vi "RT Loop - RSI Low Speed.vi"(11 "Message Queue":refnum<queue>) -> ()   [LabVIEW 2017]
doc: "This RSI Low Speed Loop VI acquires temperature data and digital inputs, and updates digital outputs."
uses:
  support/Message Queue/Message Cluster.ctl
  <vilib>/Platform/TimedLoop/XDataNode/timing_clust.ctl
  <vilib>/Platform/TimedLoop/XDataNode/nitl_modes.ctl
  <vilib>/Platform/TimedLoop/XDataNode/wakeup.ctl
  controls/Control State.ctl
  <vilib>/Platform/TimedLoop/XDataNode/loadnilvce.vi
  <vilib>/Platform/TimedLoop/XDataNode/XDataNode.xnode
  <vilib>/Platform/TimedLoop/XDataNode/XDNodeRunTimeDep.lvlib
  support/Message Queue/Message Queue.lvlib
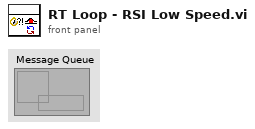
[diagram p1: front panel]
types:
  T1 = typedef "XDNodeRunTimeDep.lvlib/timing_clust.ctl" = cluster{"Expected End [f-1]":u64, "Actual End [f-1]":u64, "Finished Late? [f-1]":bool, "Expected End [i-1]":u64, "Actual End [i-1]":u64, "Finished Late? [i-1]":bool, "Expected Start [i]":u64, "Actual Start [i]":u64, "Expected Start [f]":u64, "Actual Start [f]":u64, "Source Name":string, "Structure Name":string, "Period":i64, "Deadline":i64, "Offset":i64, "Start":i64, "Priority":i32, "Timeout":i32, "Mode":T2, "Wakeup Reason":T3, "Error":errorcluster, "Source Type":string, "Secondary Source Type":string, "Global End Time":u64, "Global Start Time":u64, "Frame Duration":u64, "Iteration Duration":u64, "Assigned CPU":i32, "I/O Scan Engine Mode":u32}
  T2 = typedef "XDNodeRunTimeDep.lvlib/nitl_modes.ctl" = enum32{"No Change", "Process missed periods, maintain original phase", "Discard missed periods, maintain original phase", "Process missed periods, ignore original phase", "Discard missed periods, ignore original phase"}
  T3 = typedef "XDNodeRunTimeDep.lvlib/wakeup.ctl" = enum32{"Normal", "Aborted", "Asynchronous wakeup", "Timing source error", "Timed loop error", "Timeout"}
  T4 = typedef "Control State.ctl" = enum16{"Safe State", "Control (PID)"}
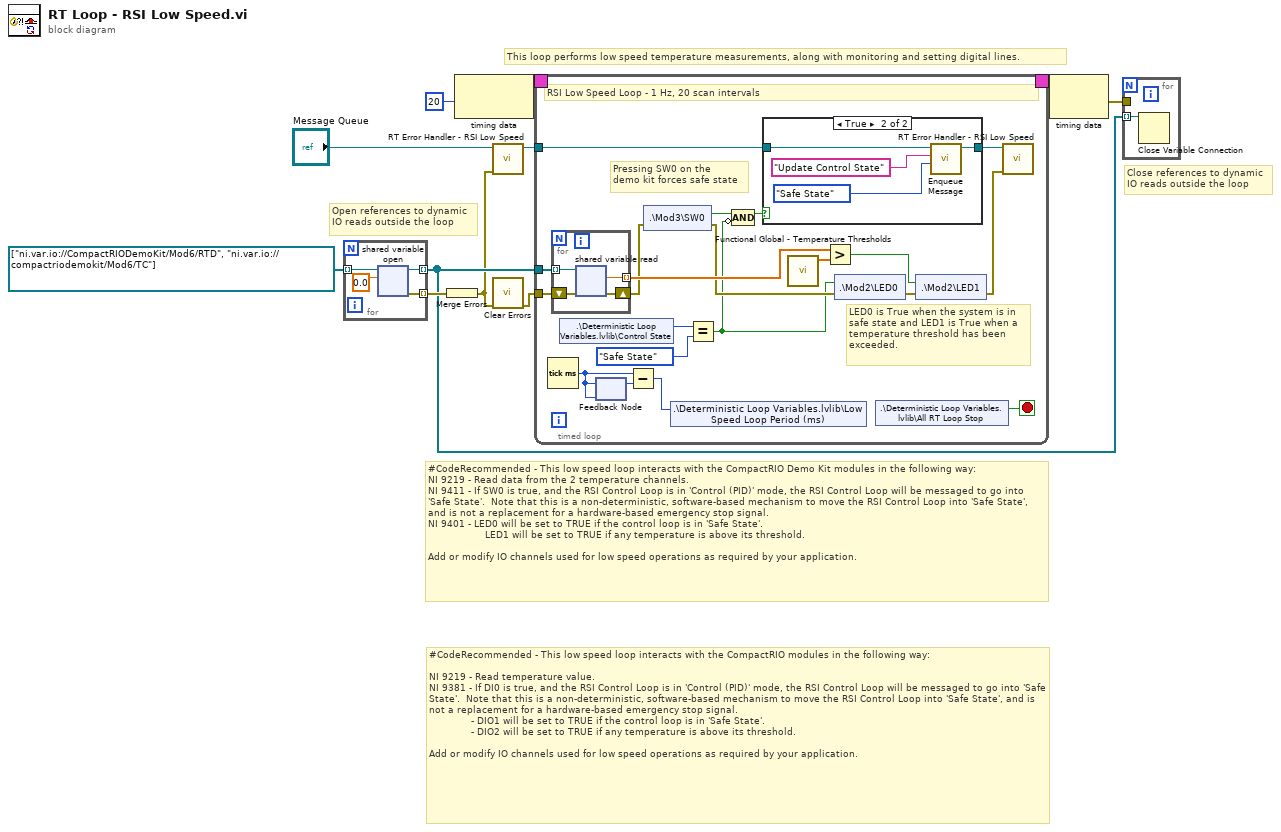
[diagram p0: block diagram]
diagram:
  # "#CodeRecommended - This low speed loop interacts with the CompactRIO modules in the following way:\n\nNI 9219 - Read temperature value.\nNI 9381 - If DI0 is true, and the RSI Control Loop is in 'Control (PID)' mode, the RSI Control Loop will be messaged to go into 'Safe State'.  Note that this is a non-deterministic, software-based mechanism to move the RSI Control Loop into 'Safe State', and is not a replacement for a hardware-based emergency stop signal.\n              - DIO1 will be set to TRUE if the control loop is in 'Safe State'.\n              - DIO2 will be set to TRUE if any temperature is above its threshold.\n\nAdd or modify IO channels used for low speed operations as required by your application."
  # "Close references to dynamic IO reads outside the loop"
  # "Open references to dynamic IO reads outside the loop"
  # "#CodeRecommended - This low speed loop interacts with the CompactRIO Demo Kit modules in the following way:\nNI 9219 - Read data from the 2 temperature channels.\nNI 9411 - If SW0 is true, and the RSI Control Loop is in 'Control (PID)' mode, the RSI Control Loop will be messaged to go into 'Safe State'.  Note that this is a non-deterministic, software-based mechanism to move the RSI Control Loop into 'Safe State', and is not a replacement for a hardware-based emergency stop signal.\nNI 9401 - LED0 will be set to TRUE if the control loop is in 'Safe State'.\n                   LED1 will be set to TRUE if any temperature is above its threshold.\n\nAdd or modify IO channels used for low speed operations as required by your application."
  # "This loop performs low speed temperature measurements, along with monitoring and setting digital lines."
  n1 = for {
    tunnel: refnum<k21>[] ["ni.var.io://CompactRIODemoKit/Mod6/RTD", "ni.var.io://compactriodemokit/Mod6/TC"] -> [w15] mode=indexing
    tunnel: [w14] -> w5 mode=indexing
    tunnel: [w12] -> w7 mode=indexing
    n2 = shared-variable-open(w15, 0.0) -> (w14:refnum<k21>, w12:errorcluster)  [unwired: 2 in]
  }
  n3 = Merge Errors(w7) -> (w3:errorcluster)
  n4 = node-c288(i64 20 ("Period")) -> (w11:T1)
  n5 = call "RT Error Handler - RSI Low Speed.vi"("error in (no error)"=w3, "Message Queue"="Message Queue") -> ("dup Message Queue"=w8:refnum<queue>)  [unwired: 8 in, 1 out]
  n6 = call <vilib>:"Clear Errors.vi"("error in (no error)"=w3) -> ("error out"=w2:errorcluster)  [unwired: 5 in, 1 out]
  n7 = timed-loop {
    timing: w11 -> [_]
    timing-out: [_] -> w10
    tunnel: w8 -> [w33]
    tunnel: w5 -> [w24]
    tunnel: w2 -> [w19]
    stop <- w18 stop-if-true
    # "Pressing SW0 on the \ndemo kit forces safe state"
    # "LED0 is True when the system is in\nsafe state and LED1 is True when a\ntemperature threshold has been \nexceeded."
    # "RSI Low Speed Loop - 1 Hz, 20 scan intervals"
    n8 = Tick Count (ms)() -> (millisecond timer value=w35:u32)
    n9 = for {
      tunnel: [w44] -> w26 mode=indexing
      tunnel: w24 -> [w43] mode=indexing
      shift-right: [w42] -> w23
      shift-left: w19 -> [w41]
      n10 = shared-variable-read(w43, w41) -> (w42:errorcluster, w44:dbl)  [unwired: 2 out]
    }
    n11 = shared-variable ".\\Deterministic Loop Variables.lvlib\\Control State"() -> (w16:T4)  [unwired: 1 in, 1 out]
    n12 = feedback #1(w35) -> (w34:u32)
    n13 = feedback-in #1(w35) -> ()
    n14 = Subtract(x=w35, y=w34) -> (x-y=w17:u32)
    n15 = shared-variable ".\\Mod3\\SW0"(error in=w23) -> (w32:bool, error out=w22:errorcluster)
    n16 = shared-variable ".\\Deterministic Loop Variables.lvlib\\Low Speed Loop Period (ms)"(w17) -> ()  [unwired: 1 in, 1 out]
    n17 = Equal?(x=w16, y=Control_State."Safe State" ("FPGA State")) -> (x = y?=w20:bool)
    n18 = Compound Arithmetic op=AND(w32, invert w20) -> (w21:bool)
    n19 = case shown="True" w21 {
      tunnel: w33 -> [w36 w40]
      tunnel: [w36 w39] -> w31
      frame False {
      }
      frame True {
        n20 = call "Enqueue Message.vi"("Message Data"=Control_State."Safe State" ("FPGA State"), "Message"="Update Control State", "Message Queue"=w40) -> ("dup Message Queue"=w39:refnum<queue>)  [unwired: 7 in, 1 out]
      }
    }
    n21 = call "Functional Global - Temperature Thresholds.vi"() -> ("Temperature Thresholds out"=w27:dbl[])  [unwired: 11 in]
    n22 = Greater?(x=w26, y=w27) -> (0:w25:bool)
    n23 = shared-variable ".\\Mod2\\LED0"(w20, error in=w22) -> (error out=w29:errorcluster)
    n24 = shared-variable ".\\Deterministic Loop Variables.lvlib\\All RT Loop Stop"() -> (w18:bool)  [unwired: 1 in, 1 out]
    n25 = shared-variable ".\\Mod2\\LED1"(w25, error in=w29) -> (error out=w28:errorcluster)
    n26 = call "RT Error Handler - RSI Low Speed.vi"("error in (no error)"=w28, "Message Queue"=w31) -> ()  [unwired: 8 in, 2 out]
  }
  n27 = node-c288(w10) -> (w6:errorcluster)
  n28 = for {
    tunnel: w6 -> [_]
    tunnel: w5 -> [w47] mode=indexing
    n29 = Close Variable Connection(11:w47) -> ()  [unwired: 1 in, 1 out]
  }
